vi "Camera Start Connected Loops.vi"   [LabVIEW 2025]
types:
  T1 = typedef "Event Setup Types.ctl" = enum16{"Default", "Camera Loop Started", "GreyScale", "Reset Camera Settings", "Reset Team Number", "Save Data", "Setting Changed", "Update Video Mode", "Video Mode Changed", "Exit"}
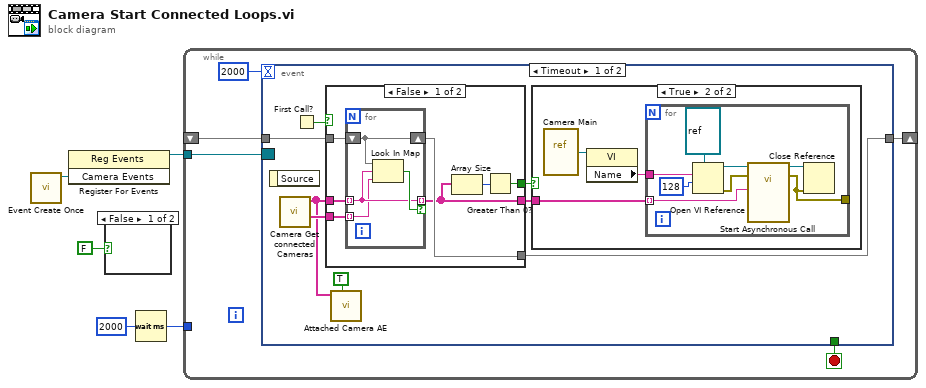
[diagram p0: block diagram]
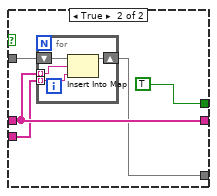
[diagram p2: hidden frame]
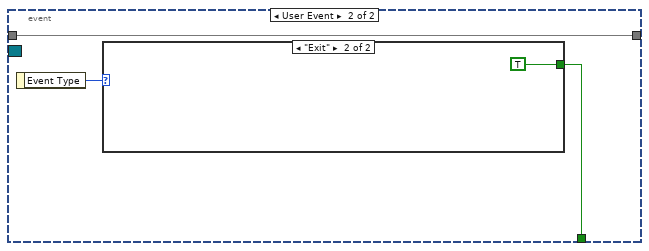
[diagram p4: hidden frame]
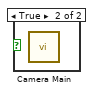
[diagram p6: hidden frame]
diagram:
  n1 = call "Event Create Once.vi"() -> ("Camera Events"=w4:refnum<user-event>)  [unwired: 10 in, 1 out]
  n2 = register-events(w4) -> (reference out=w3:refnum<event-registration>)  [unwired: 2 in, 1 out]
  n3 = case shown="False" FALSE {
    frame False {
    }
    frame True {
      n4 = call "Camera Main.vi"() -> ()  [unwired: 12 in]
    }
  }
  n5 = Wait (ms)(milliseconds to wait=u32 2000) -> (millisecond timer value=w2:u32)
  n6 = while {
    shift-right: [w9] -> _
    shift-left: _ -> [w10]
    tunnel: w3 -> [w8]
    tunnel: w2 -> [_]
    stop <- w7 stop-if-true
    n7 = event shown="[0] Timeout" {
      selector: w8 -> [_ _]
      dyn-events: _ -> [_ _]
      timeout: u32 2000 ("milliseconds to wait") -> [_ _]
      tunnel: w10 -> [w18 w50]
      tunnel: [w15 w50] -> w9
      tunnel: [_ w51] -> w7
      event Timeout {
        n8 = event-data() -> ()  [unwired: 1 in, 1 out]
        n9 = call "Camera Get connected Cameras.vi"() -> ("Product"=w13:string[], "Camera List"=w12:string[])  [unwired: 10 in]
        n10 = First Call?() -> (First Call?: T/F=w17:bool)
        n11 = case shown="False" w17 {
          tunnel: w18 -> [w25 w33]
          tunnel: w12 -> [w24 w34]
          tunnel: [w22 w34] -> w16
          tunnel: [w23 w32] -> w15
          tunnel: [w21 TRUE] -> w14
          tunnel: w13 -> [w19 w30]
          frame False {
            n12 = for {
              tunnel: w24 -> [w27] mode=indexing
              tunnel: [w27] -> w22 mode=indexing if=w28
              shift-right: [w29] -> w23
              shift-left: w25 -> [w29]
              tunnel: w19 -> [w26] mode=indexing
              n13 = Look In Map(map=w29, key=w27, default value=w26) -> (key not found?=w28:bool)  [unwired: 1 out]
            }
            n14 = Array Size(array=w22) -> (size(s)=w20:i32)
            n15 = Greater Than 0?(x=w20) -> (x > 0?=w21:bool)
          }
          frame True {
            n16 = for {
              tunnel: w34 -> [w36] mode=indexing
              shift-right: [w38] -> w32
              shift-left: w33 -> [w37]
              tunnel: w30 -> [w35] mode=indexing
              n17 = Insert Into Map(map in=w37, key=w36, value=w35) -> (map out=w38:map{string, string})  [unwired: 2 out]
            }
          }
        }
        n18 = call "Attached Camera AE.vi"("Update"=TRUE, "Camera List in"=w12) -> ()  [unwired: 9 in, 1 out]
        n19 = case shown="True" w14 {
          tunnel: w16 -> [_ w39]
          frame False {
          }
          frame True {
            n20 = vi-ref "Camera Main.vi"() -> (w41:refnum<vi>)
            n21 = property class="VI"(reference=w41) -> ("Name"=w40:string)  [unwired: 1 in, 2 out]
            n22 = for {
              tunnel: w39 -> [w43] mode=indexing
              tunnel: w40 -> [w48]
              tunnel: [w42] -> _
              n23 = Open VI Reference(type specifier VI Refnum (for type only)=refnum<vi> refnum, vi path=w48, options=128) -> (vi reference=w47:refnum<vi>, error out=w45:errorcluster)  [unwired: 3 in]
              n24 = call-by-ref "Start Asynchronous Call"(reference=w47, error in=w45, "Camera Name"=w43) -> (reference out=w46:refnum<vi>, error out=w42:errorcluster)  [unwired: 11 in]
              n25 = Close Reference(reference=w46, error in (no error)=w42) -> ()  [unwired: 1 out]
            }
          }
        }
      }
      event User Event {
        n26 = event-data() -> ("Event Type"=w52:T1)  [unwired: 1 in]
        n27 = case shown="\"Exit\"" w52 {
          tunnel: [_ TRUE] -> w51
          frame Default {
          }
          frame "Exit" {
          }
        }
      }
    }
  }
